vi "Example - Basic IPS-SA.vi"(0 "Connection Details":T5={"VISA resource name"="", "Comms Layer"=enum."Ethernet TCP/IP", "IP Address"="130.49.180.101", "Serial Configuration"={"Baud Rate"=9600, "Parity"=0, "Data Bits"=8, "Stop Bits"=10, "Flow Control"=0}, "ISOBUS address"=-1} {"Serial Configuration"."Flow Control" items=["None", "XON/XOFF", "RTS/CTS", "XON/XOFF & RTS/CTS", "DTR/DSR", "XON/XOFF & DTR/DSR"]; "Serial Configuration"."Stop Bits" items=["1.0"=10, "2.0"=20]; "Serial Configuration"."Data Bits" items=["7"=7, "8"=8]; "Serial Configuration"."Parity" items=["None", "Odd", "Even"]; "Serial Configuration"."Baud Rate" items=["300"=300, "600"=600, "1200"=1200, "2400"=2400, "4800"=4800, "9600"=9600, "19200"=19200]}, 1 "Axis Group":string(combo)="GRPZ", 2 "ID Query (True)":bool=TRUE, 3 "Clear Previous Connections (False)":bool, 4 "stop":bool, 6 "Ramp Controls":T7 {"Target Rate (T/min)" format="%_5g"; "Target Field (T)" format="%_5g"; "Target Rate (A/min)" format="%_5g"; "Target Current (A)" format="%_5g"}, 7 "AMP/TESLA":bool, 8 "Magnet Controls":T8, 9 "SWITCH\nHEATER":bool, 11 "Sw Delay (s)":dbl=30.0 caption="Time Target (s)") -> (10 "System Time":string, 12 "Device Details":T1, 13 "SW HTR\nCONFIRM":bool, 14 "Output Current (A)":dbl format="%.4g", 15 "Magnet Current (A)":dbl format="%.4g", 16 "Output Voltage (V)":dbl format="%.4g", 17 "Current/Field (A/T)":dbl caption="Current Field Factor (A/T)" format="%#.4f", 18 "PSU Act Stat 2":T9 caption="Mode Status", 19 "error out":errorcluster)   [LabVIEW 2013]
uses:
  <instrlib>/Mercury iXX/Public/Controls/Comms Transport Layer.ctl
  <instrlib>/Mercury iXX/Public/Controls/Serial Settings.ctl
  <instrlib>/Mercury iXX/Public/Controls/ISOBus Address.ctl
  <instrlib>/Mercury iXX/Public/Libraries/Magnet/Controls/Output Configuration.ctl
  <instrlib>/Mercury iXX/Public/Libraries/Magnet/Controls/PSU Actions.ctl
  <instrlib>/Mercury iXX/Public/Libraries/Magnet/Controls/Switch Heater.ctl
  <instrlib>/Mercury iXX/Public/Libraries/System/Open/Open System.vi
  <instrlib>/Mercury iXX/Public/Libraries/System/Read/Catalogue (Read).vi
  <instrlib>/Mercury iXX/Public/Libraries/Magnet/Open/Open Magnet Device.vi
  <instrlib>/Mercury iXX/Public/Libraries/Magnet/Configuration/Read/Output Configuration (Read).vi
  <instrlib>/Mercury iXX/Public/Libraries/Magnet/Configuration/Read/Current to Field Factor (Read).vi
  <instrlib>/Mercury iXX/Public/Libraries/Magnet/Configuration/Read/PSU Action Status (Read).vi
  <instrlib>/Mercury iXX/Public/Libraries/Magnet/Signals/Read/Switch Heater Status (Read).vi
  <instrlib>/Mercury iXX/Public/Libraries/Magnet/Signals/Read/Current (Read).vi
  <instrlib>/Mercury iXX/Public/Libraries/Magnet/Signals/Read/Voltage (Read).vi
  <instrlib>/Mercury iXX/Public/Libraries/Magnet/Signals/Read/Persistant Current (Read).vi
  <instrlib>/Mercury iXX/Public/Libraries/System/Read/Time (Read).vi
  <instrlib>/Mercury iXX/Public/Libraries/Magnet/Configuration/Set/PSU Action Status (Set).vi
  <instrlib>/Mercury iXX/Public/Libraries/Magnet/Signals/Set/Switch Heater No Check (Set).vi
  <instrlib>/Mercury iXX/Public/Libraries/Magnet/Signals/Set/Target Current (Set).vi
  <instrlib>/Mercury iXX/Public/Libraries/Magnet/Signals/Set/Target Current Rate (Set).vi
  <instrlib>/Mercury iXX/Public/Libraries/Magnet/Signals/Set/Target Field (Set).vi
  <instrlib>/Mercury iXX/Public/Libraries/Magnet/Signals/Set/Target Field Rate (Set).vi
  <instrlib>/Mercury iXX/Mercury iXX.lvlib
  <instrlib>/Mercury iXX/Public/Libraries/Magnet.lvlib
  <instrlib>/Mercury iXX/Public/Libraries/System.lvlib
panel:
  out "Switch Time":string
  out "Sentinel":bool
  in  "Tab Control":enum32{"Connection", "Front_Panel", "Error"}(tab)
  out "Number of Mag Units\nin the group":dbl
  out "Out Config 2":T6="PARA" caption="Output Configuration"
  out "Voltage (V)":dbl(knob) scale=-10.0..10.0
  out "Current (A)":dbl(knob) scale=-180.0..180.0
  out "Elapsed\nTime (s)":dbl caption="Elapsed Time (s)"
  out "Magnet Centre Field (T)":dbl format="%.4g"
  out "Output (T) (Field equivalent)":dbl format="%.4g"
  # "SWITCH CONTROLS"
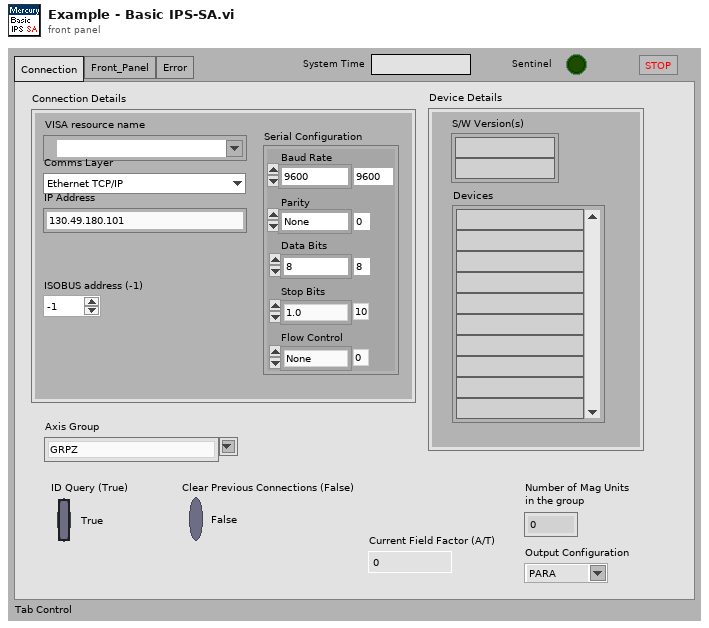
[diagram p1: front panel]
types:
  T1 = cluster{"Devices":string[], "S/W Version(s)":string[]}
  T2 = typedef "Mercury iXX.lvlib/Comms Transport Layer.ctl" = enum16{"Ethernet TCP/IP", "USB", "ISOBus - RS-232", "GPIB"}
  T3 = typedef "Mercury iXX.lvlib/Serial Settings.ctl" = cluster{"Baud Rate":u32, "Parity":u16, "Data Bits":u16, "Stop Bits":u16, "Flow Control":u16}
  T4 = typedef "Mercury iXX.lvlib/ISOBus Address.ctl" = i32
  T5 = cluster{"VISA resource name":refnum<visa-resource-name>, "Comms Layer":T2, "IP Address":string, "Serial Configuration":T3, "ISOBUS address":T4}
  T6 = typedef "Mercury iXX.lvlib/Magnet.lvlib/Output Configuration.ctl" = string
  T7 = cluster{"Target Current (A)":dbl, "Target Rate (A/min)":dbl, "SEND TO IPS":bool, "Target Field (T)":dbl, "Target Rate (T/min)":dbl}
  T8 = cluster{"CLAMP":bool, "HOLD":bool, "TO SET":bool, "TO ZERO":bool}
  T9 = typedef "Mercury iXX.lvlib/Magnet.lvlib/PSU Actions.ctl" = string
  T10 = typedef "Mercury iXX.lvlib/Mercury Reference.ctl" = cluster{"Comms":refnum<visa-resource-name>, "Device ID":string[], "Comms Layer":T2, "Command":string, "Query reference":T11}
  T11 = typedef "Mercury iXX.lvlib/Query Dynamic Reference.ctl" = refnum<vi>
  T12 = typedef "Mercury iXX.lvlib/Magnet.lvlib/Switch Heater.ctl" = string
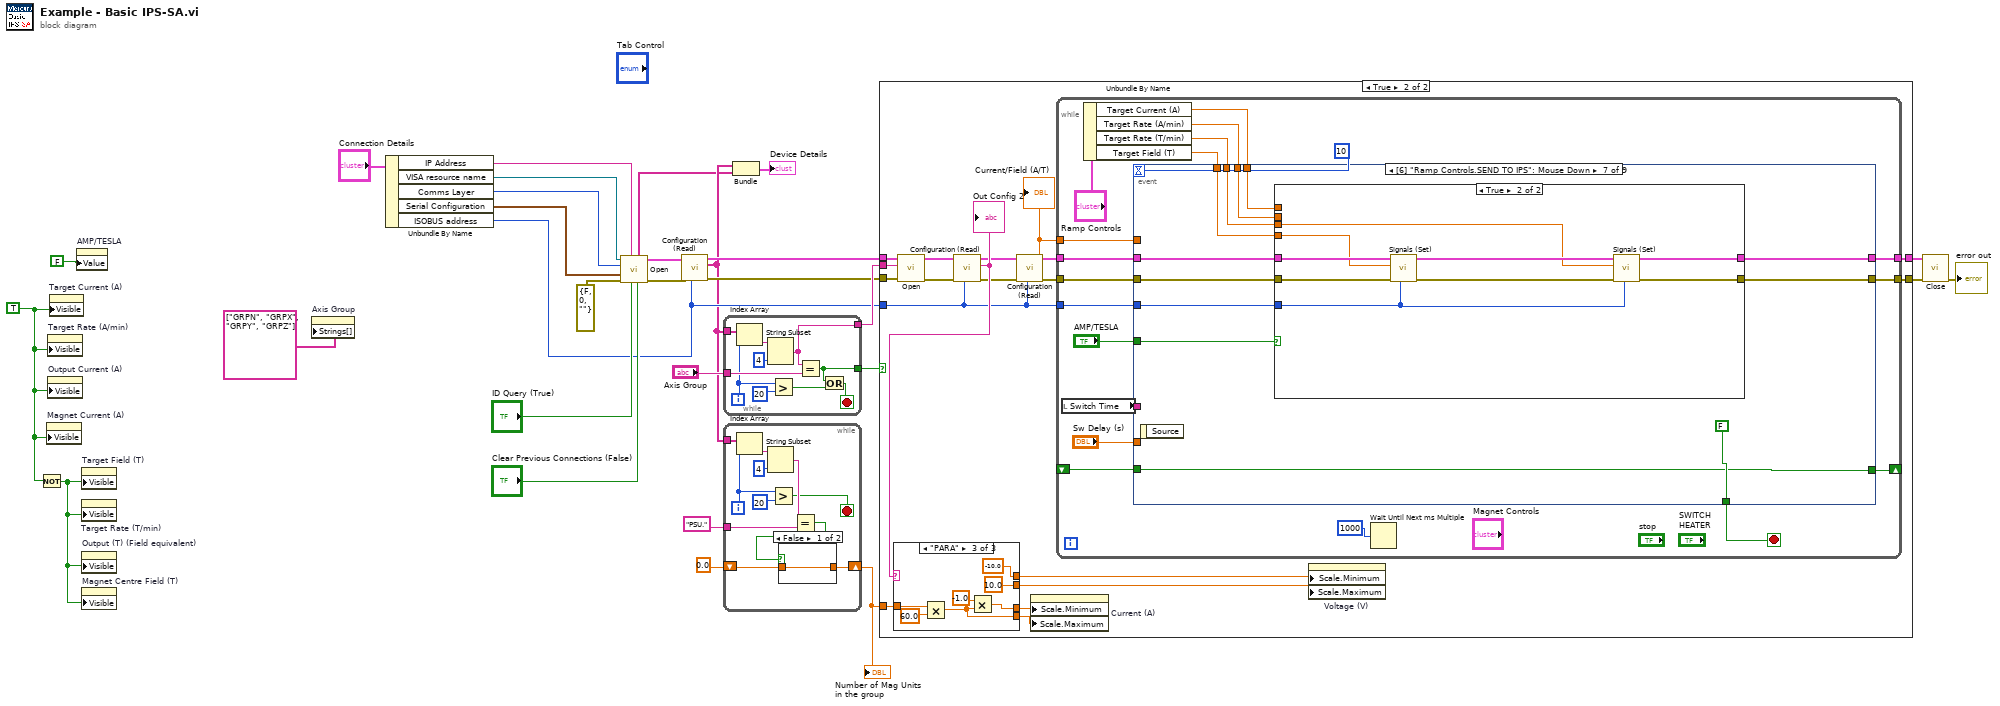
[diagram p0: block diagram]
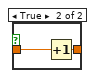
[diagram p2: hidden frame]
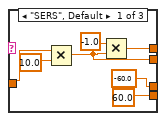
[diagram p4: hidden frame]
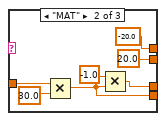
[diagram p5: hidden frame]
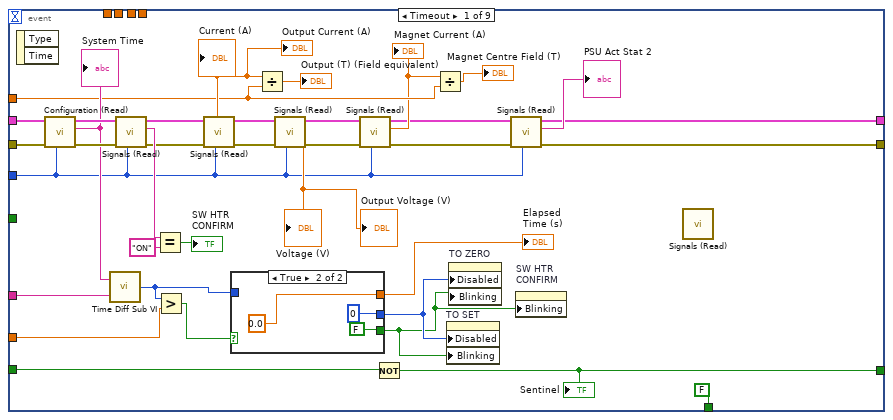
[diagram p6: hidden frame]
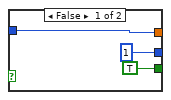
[diagram p7: hidden frame]
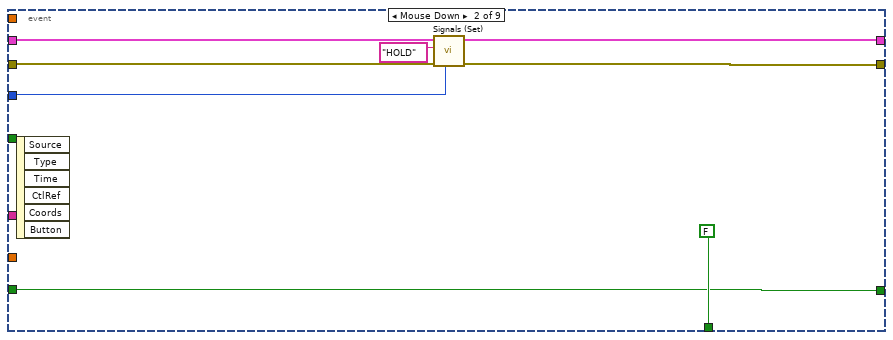
[diagram p8: hidden frame]
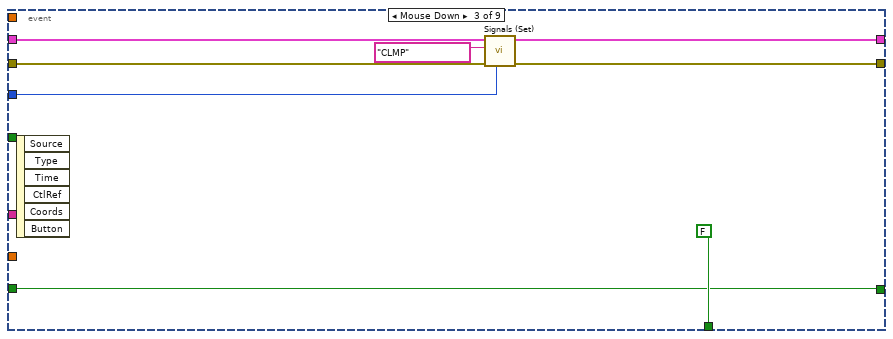
[diagram p9: hidden frame]
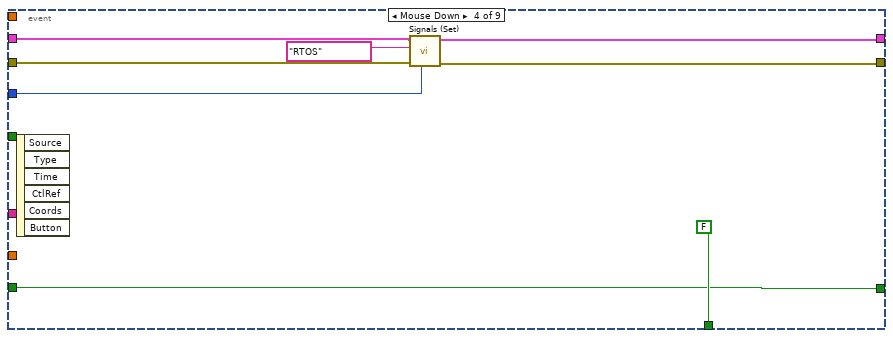
[diagram p10: hidden frame]
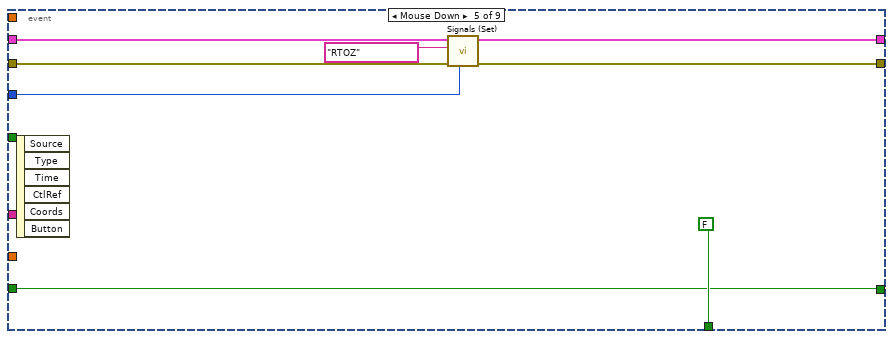
[diagram p11: hidden frame]
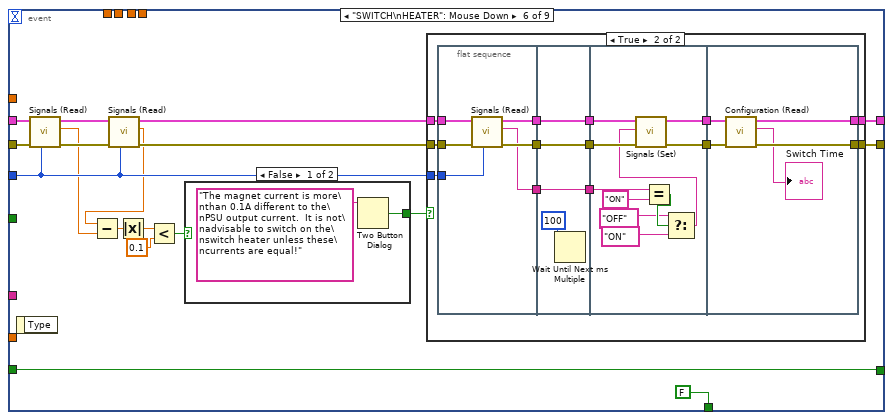
[diagram p12: hidden frame]
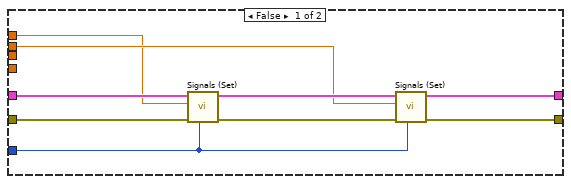
[diagram p15: hidden frame]
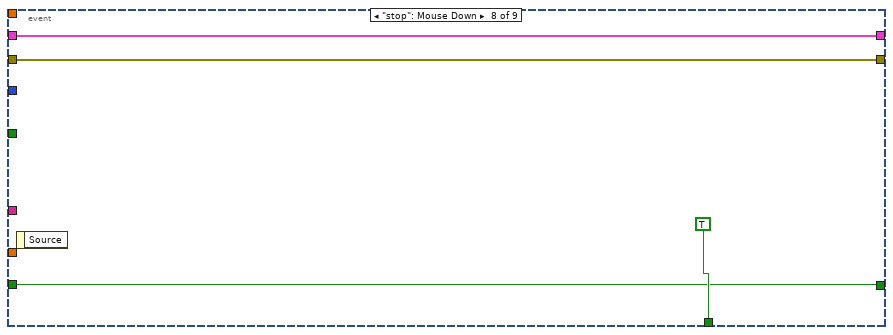
[diagram p16: hidden frame]
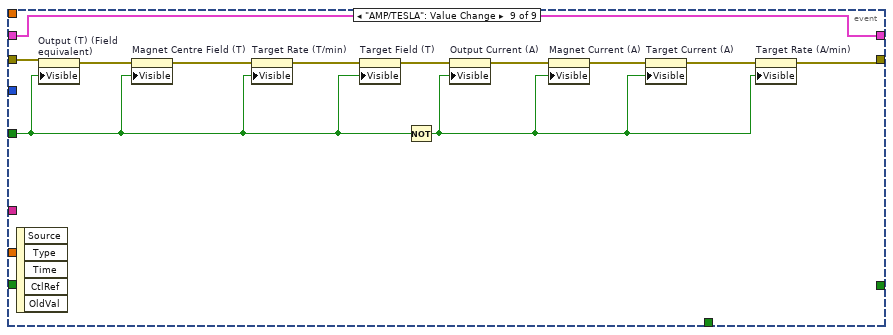
[diagram p17: hidden frame]
diagram:
  w11 = TRUE ("Visible")
  n1 = Not(x=w11) -> (.not. x?=w10:bool)
  n2 = property on="Magnet Current (A)" class="DigNum (strict)"("Visible"=w11) -> ()  [unwired: 2 in, 2 out]
  n3 = property on="Target Rate (A/min)" class="DigNum (strict)"("Visible"=w11) -> ()  [unwired: 2 in, 2 out]
  n4 = property on="Output Current (A)" class="DigNum (strict)"("Visible"=w11) -> ()  [unwired: 2 in, 2 out]
  n5 = property on="Target Current (A)" class="DigNum (strict)"("Visible"=w11) -> ()  [unwired: 2 in, 2 out]
  n6 = property on="AMP/TESLA" class="Bool (strict)"("Value"=FALSE ("AMP/TESLA")) -> ()  [unwired: 2 in, 2 out]
  n7 = property on="Target Field (T)" class="DigNum (strict)"("Visible"=w10) -> ()  [unwired: 2 in, 2 out]
  n8 = property on="Target Rate (T/min)" class="DigNum (strict)"("Visible"=w10) -> ()  [unwired: 2 in, 2 out]
  n9 = property on="Output (T) (Field equivalent)" class="DigNum (strict)"("Visible"=w10) -> ()  [unwired: 2 in, 2 out]
  n10 = property on="Magnet Centre Field (T)" class="DigNum (strict)"("Visible"=w10) -> ()  [unwired: 2 in, 2 out]
  n11 = property on="Axis Group" class="CmbBox"("Strings[]"=string[] ["GRPN", "GRPX", "GRPY", "GRPZ"]) -> ()  [unwired: 2 in, 2 out]
  n12 = Unbundle By Name("Connection Details") -> ("IP Address"=w6:string, "VISA resource name"=w5:refnum<visa-resource-name>, "Comms Layer"=w4:T2, "Serial Configuration"=w8:T3, "ISOBUS address"=w7:T4)
  n13 = call-poly <instrlib>:"Open.vi"("Clear Previous Connections (False)"="Clear Previous Connections (False)", "ID Query (True)"="ID Query (True)", "IP Address"=w6, "error in (no error)"=errorcluster {"status"=FALSE, "code"=0, "source"=""}, "Serial Configuration"=w8, "Comms Layer"=w4, "VISA resource name"=w5) -> ("error out"=w25:errorcluster, "Mercury Reference Out"=w26:T10, "S/W Version(s)"=w1:string[])  [unwired: 2 out]
  n14 = call-poly <instrlib>:"Configuration (Read).vi"("ISOBUS address"=w7, "error in"=w25, "Mercury Reference In"=w26) -> ("error out"=w13:errorcluster, "Devices"=w2:string[], "Mercury Reference Out"=w14:T10)  [unwired: 6 out]
  n15 = while {
    tunnel: w2 -> [w39]
    tunnel: [w30] -> w23
    tunnel: "Axis Group" -> [w36]
    tunnel: [w31] -> w24
    i -> [w34]
    stop <- w33 stop-if-true
    n16 = Index Array(array=w39, index=w34) -> (element=w37:string)
    n17 = String Subset(string=w37, length (rest)=4 ("length (rest)")) -> (substring=w30:string)  [unwired: 1 out]
    n18 = Greater?(x=w34, y=20) -> (0:w32:bool)
    n19 = Equal?(x=w30, y=w36) -> (x = y?=w31:bool)
    n20 = Or(x=w31, y=w32) -> (x .or. y?=w33:bool)
  }
  n21 = while {
    shift-right: [w46] -> w15
    shift-left: 0.0 -> [w45]
    tunnel: "PSU." -> [w42]
    tunnel: w2 -> [w41]
    i -> [w48]
    stop <- w43 stop-if-true
    n22 = Index Array(array=w41, index=w48) -> (element=w40:string)
    n23 = String Subset(string=w40, length (rest)=4 ("length (rest)")) -> (substring=w47:string)  [unwired: 1 out]
    n24 = Greater?(x=w48, y=20) -> (0:w43:bool)
    n25 = Equal?(x=w47, y=w42) -> (x = y?=w44:bool)
    n26 = case shown="False" w44 {
      tunnel: [w51 w53] -> w46
      tunnel: w45 -> [w51 w52]
      frame False {
      }
      frame True {
        n27 = Increment(x=w52) -> (x+1=w53:dbl)
      }
    }
  }
  "Number of Mag Units\nin the group" <- w15
  n28 = Bundle("Devices"=w2, "S/W Version(s)"=w1) -> (→"Device Details":T1)  [unwired: 1 out]
  n29 = case shown="True" w24 {
    tunnel: w14 -> [w55 w74]
    tunnel: w23 -> [_ w73]
    tunnel: w7 -> [_ w60]
    tunnel: [w55 w72] -> w22
    tunnel: [w54 w71] -> w21
    tunnel: w15 -> [_ w68]
    tunnel: w13 -> [w54 w57]
    frame False {
    }
    frame True {
      n30 = call-poly <instrlib>:"Open.vi"("error in (no error)"=w57, "Device Identifier"=w73, "Mercury Reference In"=w74) -> ("error out"=w69:errorcluster, "Mercury Reference Out"=w70:T10)  [unwired: 7 out]
      n31 = call-poly <instrlib>:"Configuration (Read).vi"("ISOBUS address"=w60, "error in"=w69, "Mercury Reference In"=w70) -> ("error out"=w62:errorcluster, "Out Config"=w67:T6, "Mercury Reference Out"=w61:T10)  [unwired: 6 out]
      "Out Config 2" <- w67
      n32 = case shown="\"PARA\"" w67 {
        tunnel: w68 -> [w79 w86 w95]
        tunnel: [60.0 ("y") w85 w92] -> w65
        tunnel: [-60.0 ("y") w84 w91] -> w66
        tunnel: [w78 -20.0 ("y") -10.0 ("y")] -> w64
        tunnel: [w77 20.0 ("y") 10.0 ("y")] -> w63
        frame "SERS", Default {
          n33 = Multiply(x=w79, y=10.0) -> (x*y=w77:dbl)
          n34 = Multiply(x=-1.0, y=w77) -> (x*y=w78:dbl)
        }
        frame "MAT" {
          n35 = Multiply(x=w86, y=30.0) -> (x*y=w85:dbl)
          n36 = Multiply(x=-1.0, y=w85) -> (x*y=w84:dbl)
        }
        frame "PARA" {
          n37 = Multiply(x=w95, y=60.0) -> (x*y=w92:dbl)
          n38 = Multiply(x=-1.0, y=w92) -> (x*y=w91:dbl)
        }
      }
      n39 = call-poly <instrlib>:"Configuration (Read).vi"("ISOBUS address"=w60, "error in"=w62, "Mercury Reference In"=w61) -> ("error out"=w59:errorcluster, "AtoB"=w56:dbl, "Mercury Reference Out"=w58:T10)  [unwired: 6 out]
      "Current/Field (A/T)" <- w56
      n40 = property on="Current (A)" class="Knob (strict)"("Scale.Minimum"=w66, "Scale.Maximum"=w65) -> ()  [unwired: 2 in, 2 out]
      n41 = while {
        tunnel: w58 -> [w112]
        tunnel: w59 -> [w111]
        tunnel: w60 -> [w110]
        shift-right: [w108] -> _
        shift-left: _ -> [w109]
        tunnel: [w106] -> w72
        tunnel: [w105] -> w71
        tunnel: w56 -> [w102]
        stop <- w107 stop-if-true
        n42 = local read "Switch Time"() -> (w104:string)
        n43 = Unbundle By Name("Ramp Controls") -> ("Target Current (A)"=w98:dbl, "Target Rate (A/min)"=w99:dbl, "Target Rate (T/min)"=w97:dbl, "Target Field (T)"=w96:dbl)
        n44 = event shown="[6] \"Ramp Controls.SEND TO IPS\": Mouse Down" {
          selector: _ -> [_ _ _ _ _ _ _ _ _]
          dyn-events: _ -> [_ _ _ _ _ _ _ _ _]
          timeout: 10 -> [_ _ _ _ _ _ _ _ _]
          tunnel: w112 -> [w148 w161 w170 w178 w186 w196 w259 w279 w282]
          tunnel: w111 -> [w147 w162 w169 w177 w185 w195 w258 w278 w293]
          tunnel: w110 -> [w118 w160 w166 w174 w184 w197 w257 _ _]
          tunnel: w109 -> [w136 w156 w164 w172 w180 w203 w253 w280 _]
          tunnel: [w135 w156 w164 w172 w180 w203 w253 w280 _] -> w108
          tunnel: [w116 w159 w168 w176 w183 w202 w256 w279 w282] -> w106
          tunnel: [w115 w158 w167 w175 w182 w201 w255 w278 w285] -> w105
          tunnel: [FALSE FALSE FALSE FALSE FALSE FALSE FALSE TRUE _] -> w107
          tunnel: w104 -> [w132 _ _ _ _ _ _ _ _]
          tunnel: "Sw Delay (s)" -> [w131 _ _ _ _ _ _ _ _]
          tunnel: w102 -> [w122 _ _ _ _ _ _ _ _]
          tunnel: "AMP/TESLA" -> [_ _ _ _ _ _ w252 _ w284]
          tunnel: w99 -> [_ _ _ _ _ _ w251 _ _]
          tunnel: w98 -> [_ _ _ _ _ _ w250 _ _]
          tunnel: w97 -> [_ _ _ _ _ _ w249 _ _]
          tunnel: w96 -> [_ _ _ _ _ _ w248 _ _]
          event Timeout {
            n45 = event-data() -> ()  [unwired: 3 out]
            n46 = call-poly <instrlib>:"Signals (Read).vi"("ISOBUS address"=w118, "error in"=w147, "Mercury Reference In"=w148) -> ("error out"=w140:errorcluster, "Switch Heater Status"=w146:string, "Mercury Reference Out"=w143:T10)  [unwired: 6 out]
            n47 = Equal?(x=w146, y="ON") -> (x = y?=→"SW HTR\nCONFIRM":bool)
            n48 = call-poly <instrlib>:"Signals (Read).vi"("ISOBUS address"=w118, "error in"=w140, "Mercury Reference In"=w143) -> ("error out"=w139:errorcluster, "Current"=w124:dbl, "Mercury Reference Out"=w142:T10)  [unwired: 6 out]
            "Current (A)" <- w124
            "Output Current (A)" <- w124
            n49 = Divide(x=w124, y=w122) -> (x/y=→"Output (T) (Field equivalent)":dbl)
            n50 = call-poly <instrlib>:"Signals (Read).vi"("ISOBUS address"=w118, "error in"=w139, "Mercury Reference In"=w142) -> ("error out"=w138:errorcluster, "Voltage"=→"Voltage (V)" →"Output Voltage (V)":dbl, "Mercury Reference Out"=w141:T10)  [unwired: 6 out]
            n51 = call-poly <instrlib>:"Signals (Read).vi"("ISOBUS address"=w118, "error in"=w138, "Mercury Reference In"=w141) -> ("error out"=w119:errorcluster, "Persistant Current"=w121:dbl, "Mercury Reference Out"=w120:T10)  [unwired: 6 out]
            "Magnet Current (A)" <- w121
            n52 = call-poly <instrlib>:"Configuration (Read).vi"("ISOBUS address"=w118, "error in"=w119, "Mercury Reference In"=w120) -> ("Time"=w133:string)  [unwired: 8 out]
            "System Time" <- w133
            n53 = call <instrlib>:"Time Diff Sub VI.vi"("Start Time (hh:mm:ss)"=w132, "Current Time (hh:mm:ss)"=w133) -> ("Time Diff (s)"=w128:i32)
            n54 = Greater?(x=w128, y=w131) -> (0:w130:bool)
            n55 = case shown="True" w130 {
              tunnel: [w151 0.0 ("Elapsed\nTime (s)")] -> w129
              tunnel: w128 -> [w151 _]
              tunnel: [TRUE ("Blinking") FALSE ("Blinking")] -> w126
              tunnel: [u8 1 ("Disabled") u8 0 ("Disabled")] -> w127
              frame False {
              }
              frame True {
              }
            }
            "Elapsed\nTime (s)" <- w129
            n56 = Not(x=w136) -> (.not. x?=w135:bool)
            "Sentinel" <- w135
            n57 = Divide(x=w121, y=w122) -> (x/y=→"Magnet Centre Field (T)":dbl)
            n58 = property on="TO SET" class="Bool"("Disabled"=w127, "Blinking"=w126) -> ()  [unwired: 2 in, 2 out]
            n59 = property on="TO ZERO" class="Bool"("Disabled"=w127, "Blinking"=w126) -> ()  [unwired: 2 in, 2 out]
            n60 = call-poly <instrlib>:"Signals (Read).vi"("ISOBUS address"=w118, "error in"=w119, "Mercury Reference In"=w120) -> ("error out"=w115:errorcluster, "PSU Act Stat"=→"PSU Act Stat 2":T9, "Mercury Reference Out"=w116:T10)  [unwired: 6 out]
            n61 = property on="SW HTR\nCONFIRM" class="Bool (strict)"("Blinking"=w126) -> ()  [unwired: 2 in, 2 out]
            n62 = call-poly <instrlib>:"Signals (Read).vi"() -> ()  [unwired: 3 in, 9 out]
          }
          event "Magnet Controls.HOLD": Mouse Down {
            n63 = event-data() -> ()  [unwired: 7 out]
            n64 = call-poly <instrlib>:"Signals (Set).vi"("ISOBUS address"=w160, "error in"=w162, "PSU Act Stat"=T9 "HOLD", "Mercury Reference In"=w161) -> ("error out"=w158:errorcluster, "Mercury Reference Out"=w159:T10)  [unwired: 6 out]
          }
          event "Magnet Controls.CLAMP": Mouse Down {
            n65 = event-data() -> ()  [unwired: 7 out]
            n66 = call-poly <instrlib>:"Signals (Set).vi"("ISOBUS address"=w166, "error in"=w169, "PSU Act Stat"=T9 "CLMP", "Mercury Reference In"=w170) -> ("error out"=w167:errorcluster, "Mercury Reference Out"=w168:T10)  [unwired: 6 out]
          }
          event "Magnet Controls.TO SET": Mouse Down {
            n67 = event-data() -> ()  [unwired: 7 out]
            n68 = call-poly <instrlib>:"Signals (Set).vi"("ISOBUS address"=w174, "error in"=w177, "PSU Act Stat"=T9 "RTOS", "Mercury Reference In"=w178) -> ("error out"=w175:errorcluster, "Mercury Reference Out"=w176:T10)  [unwired: 6 out]
          }
          event "Magnet Controls.TO ZERO": Mouse Down {
            n69 = event-data() -> ()  [unwired: 7 out]
            n70 = call-poly <instrlib>:"Signals (Set).vi"("ISOBUS address"=w184, "error in"=w185, "PSU Act Stat"=T9 "RTOZ", "Mercury Reference In"=w186) -> ("error out"=w182:errorcluster, "Mercury Reference Out"=w183:T10)  [unwired: 6 out]
          }
          event "SWITCH\nHEATER": Mouse Down {
            n71 = event-data() -> ()  [unwired: 2 out]
            n72 = call-poly <instrlib>:"Signals (Read).vi"("ISOBUS address"=w197, "error in"=w195, "Mercury Reference In"=w196) -> ("error out"=w198:errorcluster, "Current"=w191:dbl, "Mercury Reference Out"=w199:T10)  [unwired: 6 out]
            n73 = call-poly <instrlib>:"Signals (Read).vi"("ISOBUS address"=w197, "error in"=w198, "Mercury Reference In"=w199) -> ("error out"=w194:errorcluster, "Persistant Current"=w192:dbl, "Mercury Reference Out"=w193:T10)  [unwired: 6 out]
            n74 = Subtract(x=w192, y=w191) -> (x-y=w190:dbl)
            n75 = Absolute Value(x=w190) -> (abs(x)=w189:dbl)
            n76 = Less?(x=w189, y=0.1) -> (x < y?=w187:bool)
            n77 = case shown="False" w187 {
              selector: w187 -> [_ w207]
              tunnel: [w206 w207] -> w200
              frame False {
                n78 = Two Button Dialog(message="The magnet current is more\nthan 0.1A different to the\nPSU output current.  It is not\nadvisable to switch on the\nswitch heater unless these\ncurrents are equal!") -> (T button?=w206:bool)  [unwired: 2 out]
              }
              frame True {
              }
            }
            n79 = case shown="True" w200 {
              tunnel: w193 -> [w209 w214]
              tunnel: w194 -> [w208 w213]
              tunnel: w197 -> [_ w212]
              tunnel: [w209 w211] -> w202
              tunnel: [w208 w210] -> w201
              frame False {
              }
              frame True {
                n80 = flat-sequence {
                  tunnel: [w225] -> w222
                  tunnel: [w224] -> w221
                  tunnel: [w223] -> w220
                  tunnel: w214 -> [w228]
                  tunnel: w213 -> [w227]
                  tunnel: w212 -> [w226]
                  tunnel: w222 -> [w231]
                  tunnel: w221 -> [w230]
                  tunnel: [w231] -> w219
                  tunnel: [w230] -> w218
                  tunnel: [w229] -> w217
                  tunnel: w220 -> [w229]
                  tunnel: w219 -> [w241]
                  tunnel: w218 -> [w242]
                  tunnel: w217 -> [w239]
                  tunnel: [w236] -> w216
                  tunnel: [w237] -> w215
                  tunnel: w216 -> [w247]
                  tunnel: w215 -> [w246]
                  tunnel: [w245] -> w211
                  tunnel: [w244] -> w210
                  frame #0 {
                    n81 = call-poly <instrlib>:"Signals (Read).vi"("ISOBUS address"=w226, "error in"=w227, "Mercury Reference In"=w228) -> ("error out"=w225:errorcluster, "Switch Heater Status"=w223:string, "Mercury Reference Out"=w224:T10)  [unwired: 6 out]
                  }
                  frame #1 {
                    n82 = Wait Until Next ms Multiple(millisecond multiple=u32 100) -> ()  [unwired: 1 out]
                  }
                  frame #2 {
                    n83 = Equal?(x=w239, y="ON") -> (x = y?=w238:bool)
                    n84 = Select(t=T12 "OFF" ("Set Switch Heater"), s=w238, f=T12 "ON" ("Set Switch Heater")) -> (s? t:f=w233:T12)
                    n85 = call-poly <instrlib>:"Signals (Set).vi"("error in"=w241, "Set Switch Heater"=w233, "Mercury Reference In"=w242) -> ("error out"=w237:errorcluster, "Mercury Reference Out"=w236:T10)  [unwired: 1 in, 6 out]
                  }
                  frame #3 {
                    n86 = call-poly <instrlib>:"Configuration (Read).vi"("error in"=w246, "Mercury Reference In"=w247) -> ("error out"=w244:errorcluster, "Time"=→"Switch Time":string, "Mercury Reference Out"=w245:T10)  [unwired: 1 in, 6 out]
                  }
                }
              }
            }
          }
          event "Ramp Controls.SEND TO IPS": Mouse Down {
            n87 = event-data() -> ()  [unwired: 2 out]
            n88 = case shown="True" w252 {
              tunnel: w259 -> [w268 w277]
              tunnel: w258 -> [w267 w276]
              tunnel: w257 -> [w264 w271]
              tunnel: [w263 w273] -> w256
              tunnel: [w262 w272] -> w255
              tunnel: w251 -> [w261 _]
              tunnel: w250 -> [w260 _]
              tunnel: w249 -> [_ w270]
              tunnel: w248 -> [_ w269]
              frame False {
                n89 = call-poly <instrlib>:"Signals (Set).vi"("ISOBUS address"=w264, "error in"=w267, "Target Current"=w260, "Mercury Reference In"=w268) -> ("error out"=w265:errorcluster, "Mercury Reference Out"=w266:T10)  [unwired: 1 in, 5 out]
                n90 = call-poly <instrlib>:"Signals (Set).vi"("ISOBUS address"=w264, "error in"=w265, "Target Current Rate"=w261, "Mercury Reference In"=w266) -> ("error out"=w262:errorcluster, "Mercury Reference Out"=w263:T10)  [unwired: 1 in, 5 out]
              }
              frame True {
                n91 = call-poly <instrlib>:"Signals (Set).vi"("ISOBUS address"=w271, "error in"=w276, "Target Field"=w269, "Mercury Reference In"=w277) -> ("error out"=w274:errorcluster, "Mercury Reference Out"=w275:T10)  [unwired: 1 in, 5 out]
                n92 = call-poly <instrlib>:"Signals (Set).vi"("ISOBUS address"=w271, "error in"=w274, "Target Field Rate"=w270, "Mercury Reference In"=w275) -> ("error out"=w272:errorcluster, "Mercury Reference Out"=w273:T10)  [unwired: 1 in, 5 out]
              }
            }
          }
          event "stop": Mouse Down {
            n93 = event-data() -> ()  [unwired: 2 out]
          }
          event "AMP/TESLA": Value Change {
            n94 = event-data() -> ()  [unwired: 6 out]
            n95 = property on="Output (T) (Field equivalent)" class="DigNum (strict)"(error in=w293, "Visible"=w284) -> (error out=w292:errorcluster)  [unwired: 1 in, 1 out]
            n96 = property on="Magnet Centre Field (T)" class="DigNum (strict)"(error in=w292, "Visible"=w284) -> (error out=w291:errorcluster)  [unwired: 1 in, 1 out]
            n97 = property on="Target Rate (T/min)" class="DigNum (strict)"(error in=w291, "Visible"=w284) -> (error out=w290:errorcluster)  [unwired: 1 in, 1 out]
            n98 = property on="Target Field (T)" class="DigNum (strict)"(error in=w290, "Visible"=w284) -> (error out=w289:errorcluster)  [unwired: 1 in, 1 out]
            n99 = Not(x=w284) -> (.not. x?=w283:bool)
            n100 = property on="Output Current (A)" class="DigNum (strict)"(error in=w289, "Visible"=w283) -> (error out=w288:errorcluster)  [unwired: 1 in, 1 out]
            n101 = property on="Magnet Current (A)" class="DigNum (strict)"(error in=w288, "Visible"=w283) -> (error out=w287:errorcluster)  [unwired: 1 in, 1 out]
            n102 = property on="Target Current (A)" class="DigNum (strict)"(error in=w287, "Visible"=w283) -> (error out=w286:errorcluster)  [unwired: 1 in, 1 out]
            n103 = property on="Target Rate (A/min)" class="DigNum (strict)"(error in=w286, "Visible"=w283) -> (error out=w285:errorcluster)  [unwired: 1 in, 1 out]
          }
        }
        n104 = Wait Until Next ms Multiple(millisecond multiple=u32 1000) -> ()  [unwired: 1 out]
      }
      n105 = property on="Voltage (V)" class="Knob (strict)"("Scale.Minimum"=w64, "Scale.Maximum"=w63) -> ()  [unwired: 2 in, 2 out]
    }
  }
  n106 = call <instrlib>:"Close.vi"("error in (no error)"=w21, "Mercury Reference"=w22) -> ("error out"=→"error out":errorcluster)  [unwired: 9 out]
